vi "Result_Test.vi"(8 "error in (no error)":errorcluster caption="entrée d'erreur (pas d'erreur)", 11 "Get_Voltage en entrée":refnum<class "Zigbee_White_List.lvclass">) -> (0 "error out":errorcluster caption="sortie d'erreur", 3 "Get_Voltage en sortie":refnum<class "Zigbee_White_List.lvclass">)   [LabVIEW 2020, in "Library Test.lvlib" / "Zigbee_White_List.lvclass"]
uses:
  Zigbee_White_List.lvclass
  C:/Users/ngarcin/OneDrive - Altyor/Standard TB/Class/Test/Test (Default)/Test (Default).lvclass
  C:/Users/ngarcin/OneDrive - Altyor/Standard TB/Class/Test/Zigbee_Send_Command_UART/Zigbee_Send_Command_UART.lvclass
  Zigbee_Send_Command_UART/Zigbee_Send_Command_UART.lvclass
  Zigbee_White_List.lvclass/Zigbee_White_List.ctl
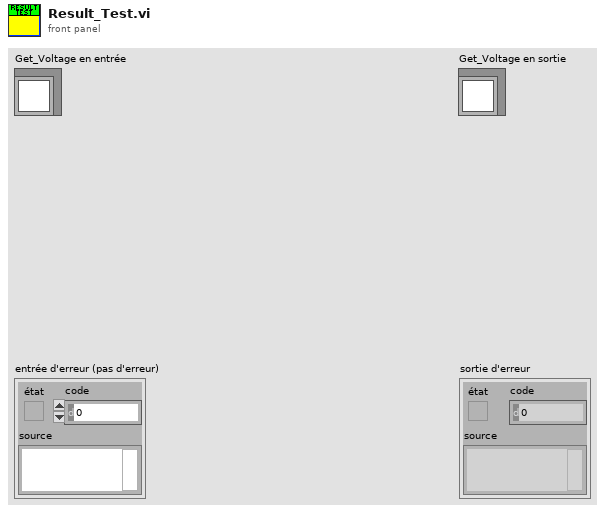
[diagram p1: front panel]
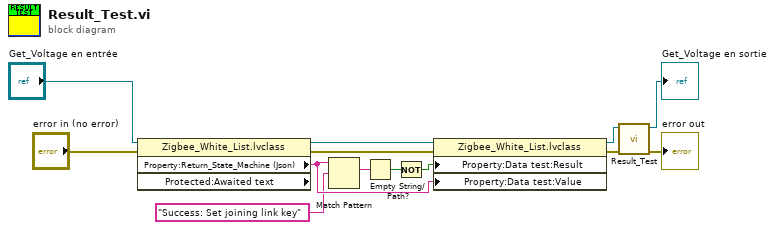
[diagram p0: block diagram]
diagram:
  n1 = property class="Zigbee_White_List.lvclass" props=["Property:Return_State_Machine (Json)", "Protected:Awaited text"](reference="Get_Voltage en entrée", error in="error in (no error)") -> (reference out=w11:refnum<class "Zigbee_White_List.lvclass">, error out=w6:errorcluster, "Property:Return_State_Machine (Json)"=w5:string)  [unwired: 1 out]
  n2 = Match Pattern(string=w5, regular expression="Success: Set joining link key" ("expression régulière")) -> (match substring=w3:string)  [unwired: 1 in, 3 out]
  n3 = Empty String/Path?(string/path=w3) -> (empty?=w2:bool)
  n4 = Not(x=w2) -> (.not. x?=w1:bool)
  n5 = property class="Zigbee_White_List.lvclass"(reference=w11, error in=w6, "Property:Data test:Result"=w1, "Property:Data test:Value"=w5) -> (reference out=w7:refnum<class "Zigbee_White_List.lvclass">, error out=w8:errorcluster)
  n6 = call-parent "Result_Test.vi"("error in (no error)"=w8, "Get_Voltage en entrée"=w7) -> ("error out"=→"error out":errorcluster, "Get_Voltage en sortie"=→"Get_Voltage en sortie":refnum<class "Zigbee_White_List.lvclass">)  [unwired: 8 in]
